vi "Speed of Light FPGA VI.vi"() -> ()   [LabVIEW 2026]
uses:
  <vilib>/rvi/Emulation/niFpgaGetClockAttributes.vi
  <vilib>/rvi/Emulation/niFpgaSctlEmulationGetInTimedLoop.vi
  <vilib>/rvi/Emulation/niFpgaEmulationReportErrorSimple.vi
  <vilib>/rvi/eio/common/nirviEmuTemplateMethod_errors.vi
  <vilib>/rvi/Emulation/niFpgaCriticalErrorInLSC.vi
  <vilib>/eio/EIONode/EIONode.xnode
panel:
  in  "LEDs start":bool[](array[boolean])=[FALSE, TRUE, FALSE, TRUE, FALSE, TRUE, FALSE, FALSE, TRUE, FALSE, FALSE, TRUE, FALSE, FALSE, FALSE, TRUE, TRUE, FALSE, FALSE, FALSE, FALSE, FALSE, FALSE, FALSE, FALSE, FALSE, FALSE, FALSE, FALSE, FALSE, FALSE, FALSE]
  out "LEDs":bool[](array[boolean])
  out "Buttons":bool[](array[boolean])
  out "Time to \nComplete (micro)":u32
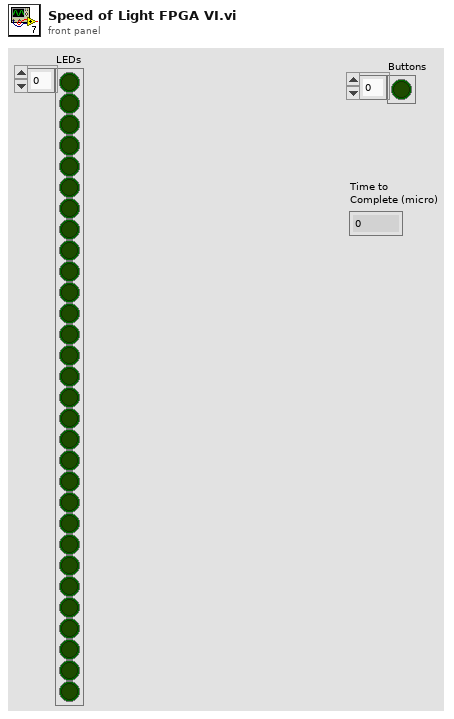
[diagram p1: front panel]
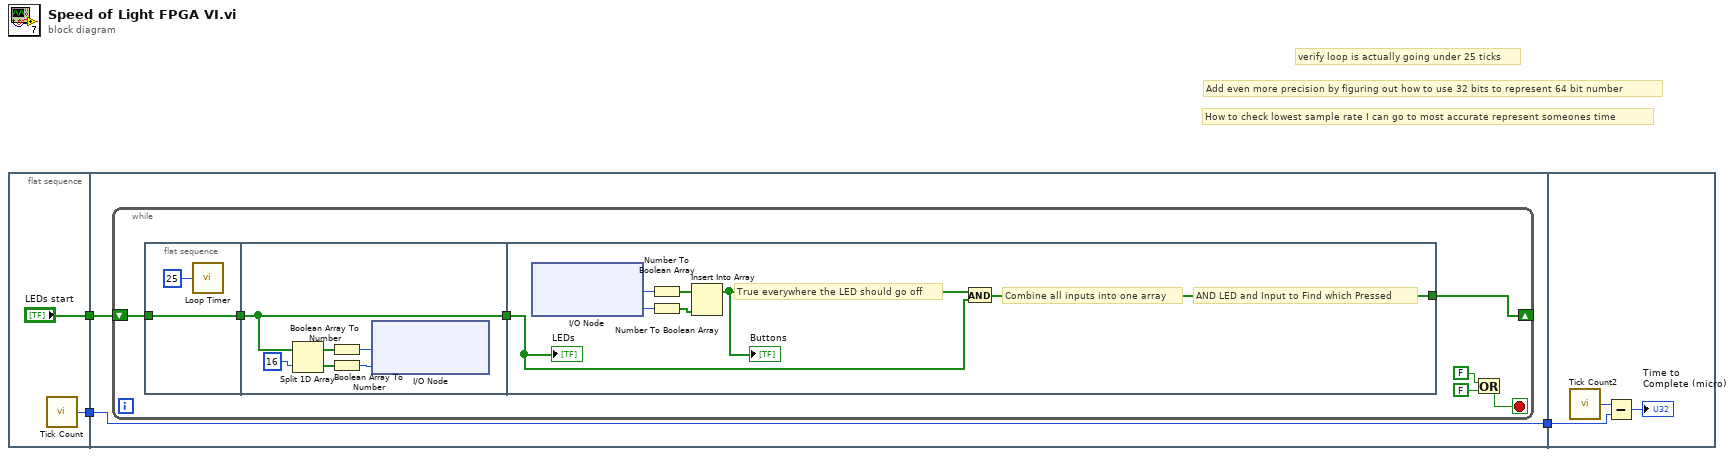
[diagram p0: block diagram]
diagram:
  # "verify loop is actually going under 25 ticks"
  # "How to check lowest sample rate I can go to most accurate represent someones time"
  # "Add even more precision by figuring out how to use 32 bits to represent 64 bit number"
  n1 = flat-sequence {
    tunnel: [w5] -> w2
    tunnel: ["LEDs start"] -> w1
    tunnel: [w7] -> w3
    tunnel: w2 -> [w7]
    tunnel: w1 -> [w6]
    tunnel: w3 -> [w32]
    frame #0 {
      n2 = call "Tick Count"() -> ("Tick Count(uSec)"=w5:u32)
    }
    frame #1 {
      n3 = while {
        shift-right: [w11] -> _
        shift-left: w6 -> [w10]
        stop <- w13 stop-if-true
        n4 = flat-sequence {
          tunnel: w10 -> [w15]
          tunnel: [w15] -> w9
          tunnel: [w17] -> w12
          tunnel: w9 -> [w17]
          tunnel: w12 -> [w23]
          tunnel: [w25] -> w11
          frame #0 {
            n5 = call "Loop Timer"("Count(uSec)"=u8 25 ("Count(Ticks)")) -> ()  [unwired: 1 out]
          }
          frame #1 {
            n6 = Split 1D Array(array=w17, index=16) -> (first subarray=w21:bool[], second subarray=w20:bool[])
            n7 = Boolean Array To Number(Boolean array=w21) -> (number=w19:u16)
            n8 = Boolean Array To Number(Boolean array=w20) -> (number=w18:u16)
            n9 = xnode "I/O Node"("Mod7/DO15:0"=w19, "Mod5/DO15:0"=w18) -> ()  [unwired: 2 in, 2 out]
          }
          frame #2 {
            # "True everywhere the LED should go off"
            # "AND LED and Input to Find which Pressed"
            # "Combine all inputs into one array"
            n10 = xnode "I/O Node"() -> ("Mod7/DI15:0"=w28:u16, "Mod5/DI15:0"=w27:u16)  [unwired: 2 in, 2 out]
            n11 = Number To Boolean Array(number=w28) -> (Boolean array=w29:bool[])
            n12 = Number To Boolean Array(number=w27) -> (Boolean array=w26:bool[])
            n13 = Insert Into Array(array=w29, new element=w26) -> (w24:bool[])  [unwired: 1 in]
            "Buttons" <- w24
            n14 = And(x=w24, y=w23) -> (x .and. y?=w25:bool[])
            "LEDs" <- w23
          }
        }
        n15 = Or(x=FALSE, y=FALSE ("stop")) -> (x .or. y?=w13:bool)
      }
    }
    frame #2 {
      n16 = call "Tick Count2"() -> ("Tick Count(uSec)"=w31:u32)
      n17 = Subtract(x=w31, y=w32) -> (x-y=→"Time to \nComplete (micro)":u32)
    }
  }
